vi "EEPROM读取模块.vi"(8 "input_array_temp_int":u8[][](array[numeric]) format="%.0x", 9 "input_str_labelType":string, 10 "VISA :":refnum<visa-resource-name>, 11 "Adaptor":enum16{"RS232 - IIC", "LUXSHARE - IIC"}(ring)) -> (2 "pagesEqual00?":bool, 3 "show_array_read_int":u8[][](array[numeric]) format="%.0x")   [LabVIEW 2011]
panel:
  out "数组":bool[](array[boolean])
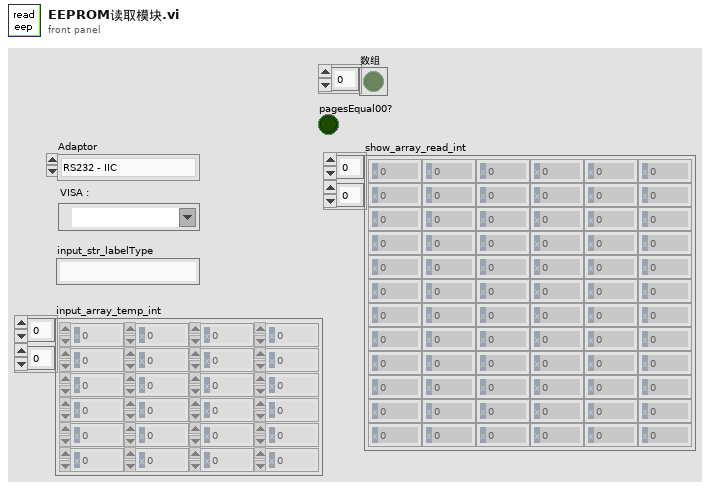
[diagram p1: front panel]
types:
  T1 = enum16{"Write to EEPROM", "Read From EEPROM", "Read From EEPROM1"}
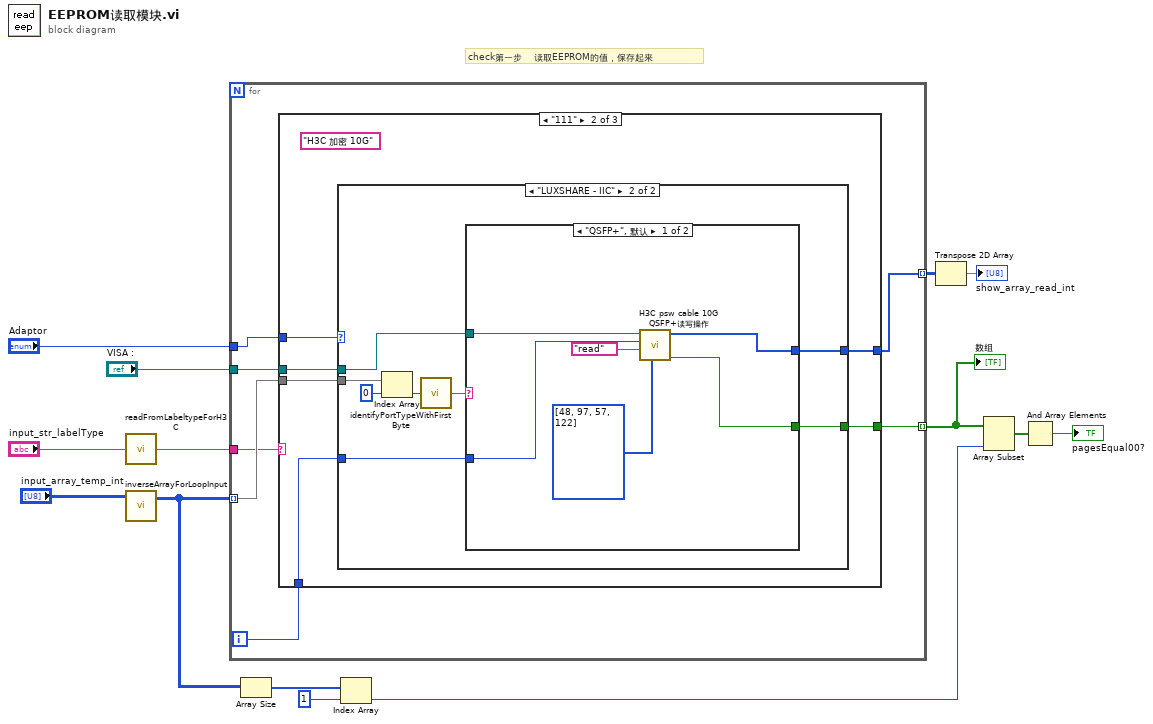
[diagram p0: block diagram]
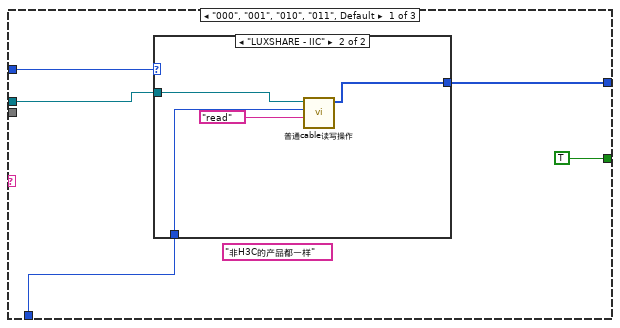
[diagram p2: hidden frame]
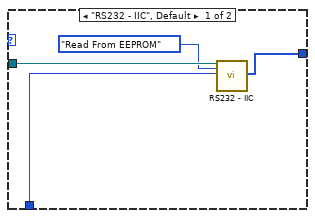
[diagram p3: hidden frame]
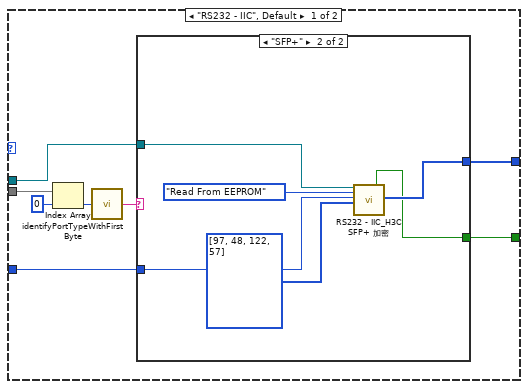
[diagram p4: hidden frame]
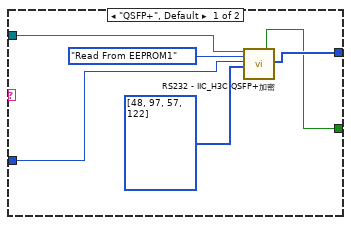
[diagram p5: hidden frame]
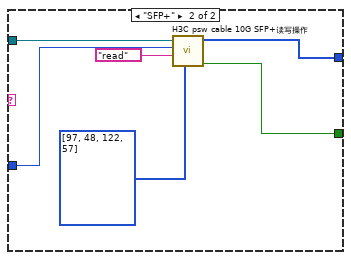
[diagram p6: hidden frame]
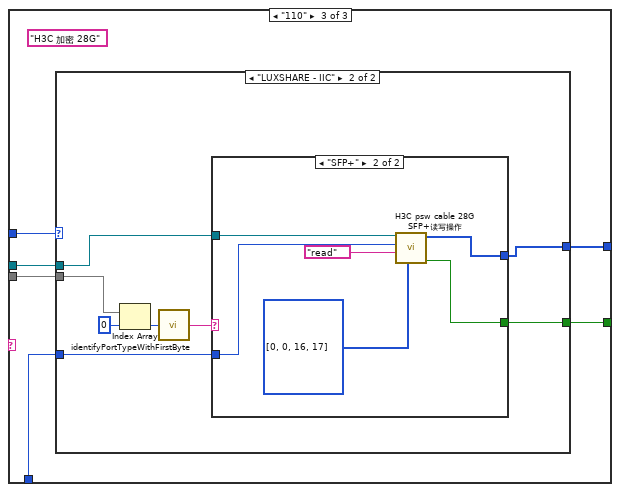
[diagram p7: hidden frame]
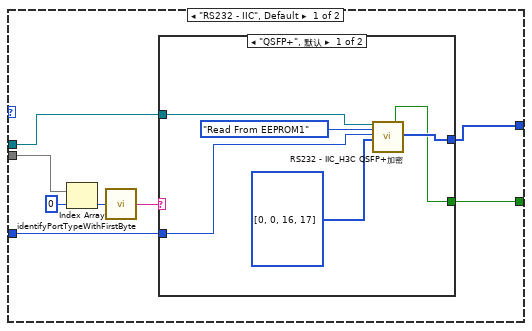
[diagram p8: hidden frame]
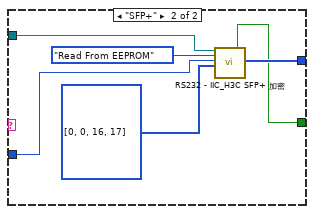
[diagram p9: hidden frame]
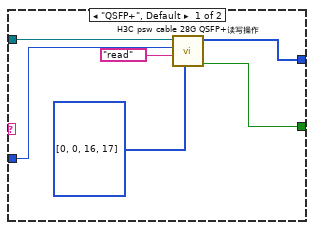
[diagram p10: hidden frame]
diagram:
  # "check第一步    读取EEPROM的值，保存起来"
  n1 = call "readFromLabeltypeForH3C.vi"("input_str_labelType"="input_str_labelType") -> ("show_str_011string"=w14:string)
  n2 = call "inverseArrayForLoopInput.vi"("input_array_temp_int"="input_array_temp_int") -> ("show_array_temp_int"=w7:u8[][])  [unwired: 1 in, 1 out]
  n3 = for {
    tunnel: "VISA :" -> [w20]
    tunnel: w7 -> [w18] mode=indexing
    tunnel: [w19] -> w9 mode=indexing
    tunnel: w14 -> [w17]
    tunnel: "Adaptor" -> [w16]
    tunnel: [w15] -> w8 mode=indexing
    i -> [w21]
    n4 = case shown="\"111\"" w17 {
      tunnel: w20 -> [w26 w40 w86]
      tunnel: w18 -> [_ w38 w84]
      tunnel: w21 -> [w25 w39 w85]
      tunnel: [w24 w37 w83] -> w19
      tunnel: w16 -> [w23 w36 w82]
      tunnel: [TRUE w35 w81] -> w15
      frame "000", "001", "010", "011", Default {
        (unwired) "非H3C的产品都一样"
        n5 = case shown="\"LUXSHARE - IIC\"" w23 {
          tunnel: w26 -> [w30 w33]
          tunnel: w25 -> [w28 w32]
          tunnel: [w27 w34] -> w24
          frame "RS232 - IIC", Default {
            n6 = call "RS232 - IIC.vi"("VISA resource name"=w30, "Function"=enum16{"Write to EEPROM", "Read From EEPROM"}."Read From EEPROM", "Select channel"=w28) -> ("Data from Read"=w27:u8[])  [unwired: 10 in, 6 out]
          }
          frame "LUXSHARE - IIC" {
            n7 = call "普通cable读写操作.vi"("input_mode"="read", "Channel"=w32, "VISA"=w33) -> ("data read"=w34:u8[])  [unwired: 7 in, 1 out]
          }
        }
      }
      frame "111" {
        (unwired) "H3C 加密 10G"
        n8 = case shown="\"LUXSHARE - IIC\"" w36 {
          tunnel: w40 -> [w45 w65]
          tunnel: w39 -> [w44 w64]
          tunnel: w38 -> [w43 w63]
          tunnel: [w42 w62] -> w37
          tunnel: [w41 w61] -> w35
          frame "RS232 - IIC", Default {
            n9 = Index Array(array=w43, index=0 ("索引")) -> (element=w47:u8)
            n10 = call "identifyPortTypeWithFirstByte.vi"("input_int"=w47) -> ("show_str_portType"=w46:string)
            n11 = case shown="\"SFP+\"" w46 {
              tunnel: w45 -> [w54 w59]
              tunnel: w44 -> [w53 w57]
              tunnel: [w52 w58] -> w42
              tunnel: [w49 w55] -> w41
              frame "QSFP+", Default {
                n12 = call "RS232 - IIC_H3C QSFP+加密.vi"("VISA resource name"=w54, "Function"=T1."Read From EEPROM1", "Select channel"=w53, "input_psw"=u8[] [48, 97, 57, 122]) -> ("3PagesEqual0"=w49:bool, "Data from Read"=w52:u8[])  [unwired: 8 in, 6 out]
              }
              frame "SFP+" {
                n13 = call "RS232 - IIC_H3C SFP+ 加密.vi"("VISA resource name"=w59, "Function"=enum16{"Write to EEPROM", "Read From EEPROM"}."Read From EEPROM", "Select channel"=w57, "psw"=u8[] [97, 48, 122, 57]) -> ("A2HEqual0"=w55:bool, "Data from Read"=w58:u8[])  [unwired: 9 in, 5 out]
              }
            }
          }
          frame "LUXSHARE - IIC" {
            n14 = Index Array(array=w63, index=0 ("索引")) -> (element=w67:u8)
            n15 = call "identifyPortTypeWithFirstByte.vi"("input_int"=w67) -> ("show_str_portType"=w66:string)
            n16 = case shown="\"QSFP+\", 默认" w66 {
              tunnel: w65 -> [w74 w80]
              tunnel: w64 -> [w73 w78]
              tunnel: [w72 w79] -> w62
              tunnel: [w70 w75] -> w61
              frame "QSFP+", Default {
                n17 = call "H3C psw cable 10G QSFP+读写操作.vi"("input_psw"=u8[] [48, 97, 57, 122], "input_mode"="read", "Channel"=w73, "VISA"=w74) -> ("123equal0?"=w70:bool, "data read"=w72:u8[])  [unwired: 4 in, 2 out]
              }
              frame "SFP+" {
                n18 = call "H3C psw cable 10G SFP+读写操作.vi"("input_psw"=u8[] [97, 48, 122, 57] ("psw"), "input_mode"="read", "Channel"=w78, "VISA"=w80) -> ("A2Hequal00?"=w75:bool, "data read"=w79:u8[])  [unwired: 4 in, 2 out]
              }
            }
          }
        }
      }
      frame "110" {
        (unwired) "H3C 加密 28G"
        n19 = case shown="\"LUXSHARE - IIC\"" w82 {
          tunnel: w86 -> [w91 w111]
          tunnel: w85 -> [w90 w110]
          tunnel: w84 -> [w89 w109]
          tunnel: [w88 w108] -> w83
          tunnel: [w87 w107] -> w81
          frame "RS232 - IIC", Default {
            n20 = Index Array(array=w89, index=0 ("索引")) -> (element=w93:u8)
            n21 = call "identifyPortTypeWithFirstByte.vi"("input_int"=w93) -> ("show_str_portType"=w92:string)
            n22 = case shown="\"QSFP+\", 默认" w92 {
              tunnel: w91 -> [w100 w105]
              tunnel: w90 -> [w99 w103]
              tunnel: [w97 w104] -> w88
              tunnel: [w95 w101] -> w87
              frame "QSFP+", Default {
                n23 = call "RS232 - IIC_H3C QSFP+加密.vi"("VISA resource name"=w100, "Function"=T1."Read From EEPROM1", "Select channel"=w99, "input_psw"=u8[] [0, 0, 16, 17]) -> ("3PagesEqual0"=w95:bool, "Data from Read"=w97:u8[])  [unwired: 8 in, 6 out]
              }
              frame "SFP+" {
                n24 = call "RS232 - IIC_H3C SFP+ 加密.vi"("VISA resource name"=w105, "Function"=enum16{"Write to EEPROM", "Read From EEPROM"}."Read From EEPROM", "Select channel"=w103, "psw"=u8[] [0, 0, 16, 17]) -> ("A2HEqual0"=w101:bool, "Data from Read"=w104:u8[])  [unwired: 9 in, 5 out]
              }
            }
          }
          frame "LUXSHARE - IIC" {
            n25 = Index Array(array=w109, index=0 ("索引")) -> (element=w113:u8)
            n26 = call "identifyPortTypeWithFirstByte.vi"("input_int"=w113) -> ("show_str_portType"=w112:string)
            n27 = case shown="\"SFP+\"" w112 {
              tunnel: w111 -> [w120 w126]
              tunnel: w110 -> [w119 w123]
              tunnel: [w117 w125] -> w108
              tunnel: [w116 w124] -> w107
              frame "QSFP+", Default {
                n28 = call "H3C psw cable 28G QSFP+读写操作.vi"("input_psw"=u8[] [0, 0, 16, 17], "input_mode"="read", "Channel"=w119, "VISA"=w120) -> ("123equal0?"=w116:bool, "data read"=w117:u8[])  [unwired: 4 in, 2 out]
              }
              frame "SFP+" {
                n29 = call "H3C psw cable 28G SFP+读写操作.vi"("input_psw"=u8[] [0, 0, 16, 17] ("psw"), "input_mode"="read", "Channel"=w123, "VISA"=w126) -> ("A2Hequal00?"=w124:bool, "data read"=w125:u8[])  [unwired: 4 in, 2 out]
              }
            }
          }
        }
      }
    }
  }
  "数组" <- w8
  n30 = Array Size(array=w7) -> (size(s)=w6:i32[])
  n31 = Index Array(array=w6, index=1 ("索引")) -> (element=w4:i32)
  n32 = Transpose 2D Array(2D array=w9) -> (transposed array=→"show_array_read_int":u8[][])
  n33 = Array Subset(array=w8, length=w4) -> (w3:bool[])  [unwired: 1 in]
  n34 = And Array Elements(Boolean array=w3) -> (logical AND=→"pagesEqual00?":bool)
